vi "未命名aaa.vi"(11 "Slide引用句柄":refnum<vi>) -> ()   [LabVIEW 2015]
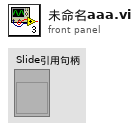
[diagram p1: front panel]
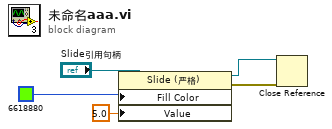
[diagram p0: block diagram]
diagram:
  n1 = property class="Slide (严格)"(reference="Slide引用句柄", "Fill Color"=u32 6618880, "Value"=5.0 ("值")) -> (reference out=w2:refnum<vi>, error out=w1:errorcluster)  [unwired: 1 in]
  n2 = Close Reference(reference=w2, error in (no error)=w1) -> ()  [unwired: 1 out]
